vi "TORC-TapeMeasureAutonomousExample.vi"   [LabVIEW 2014]
doc: "One of the VIs created by TORC 2137 to control the tape measure. Please copy this code and place it in your Autonomous Independent.vi.\n\nThis VI is an example of the usage for the Autonomous PID and Autonomous Manual within an autonomous program that utilizes Labview's \"film\" Sequence to execute commands in order."
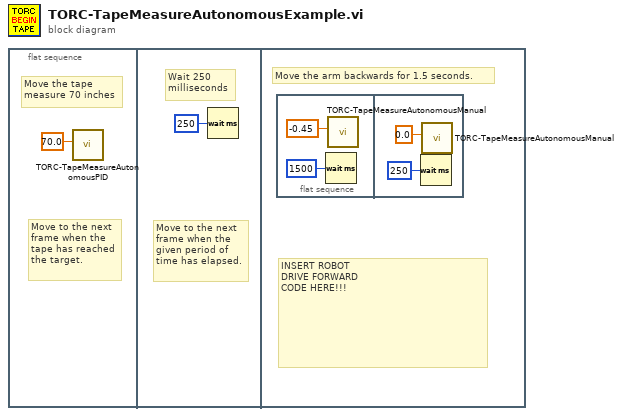
[diagram p0: block diagram]
diagram:
  n1 = flat-sequence {
    frame #0 {
      # "Move to the next\nframe when the\ntape has reached\nthe target."
      # "Move the tape\nmeasure 70 inches"
      n2 = call "TORC-TapeMeasureAutonomousPID.vi"("Target"=70.0) -> ()  [unwired: 11 in]
    }
    frame #1 {
      # "Move to the next\nframe when the\ngiven period of\ntime has elapsed."
      # "Wait 250\nmilliseconds"
      n3 = Wait (ms)(milliseconds to wait=u32 250) -> ()  [unwired: 1 out]
    }
    frame #2 {
      # "INSERT ROBOT\nDRIVE FORWARD\nCODE HERE!!!"
      # "Move the arm backwards for 1.5 seconds."
      n4 = flat-sequence {
        frame #0 {
          n5 = Wait (ms)(milliseconds to wait=u32 1500) -> ()  [unwired: 1 out]
          n6 = call "TORC-TapeMeasureAutonomousManual.vi"("Target Speed"=-0.45) -> ()  [unwired: 11 in]
        }
        frame #1 {
          n7 = Wait (ms)(milliseconds to wait=u32 250) -> ()  [unwired: 1 out]
          n8 = call "TORC-TapeMeasureAutonomousManual.vi"("Target Speed"=0.0) -> ()  [unwired: 11 in]
        }
      }
    }
  }
